vi "(Depricated) EnQ Syringe Pressure State.vi"(6 "Raw Pressure":dbl=nan, 7 "d/dt":dbl, 8 "error in (no error)":errorcluster, 9 "Pressure":dbl=nan, 10 "State":T1, 11 "cRIO Vacuum in":refnum<class "cRIO Vacuum.lvclass">) -> (0 "error out":errorcluster, 1 "overflow?":bool, 2 "Overflow State":T1, 3 "cRIO Vacuum out":refnum<class "cRIO Vacuum.lvclass">, 4 "Overflow Pressure":dbl, 5 "overflow d/dt":dbl)   [LabVIEW 2015]
uses:
  Controls/Vacuum State Enumerator.ctl
  Controls/Vacuum State Cluster.ctl
  cRIO Vacuum.lvclass
panel:
  out "Overflow Raw Pressure":dbl
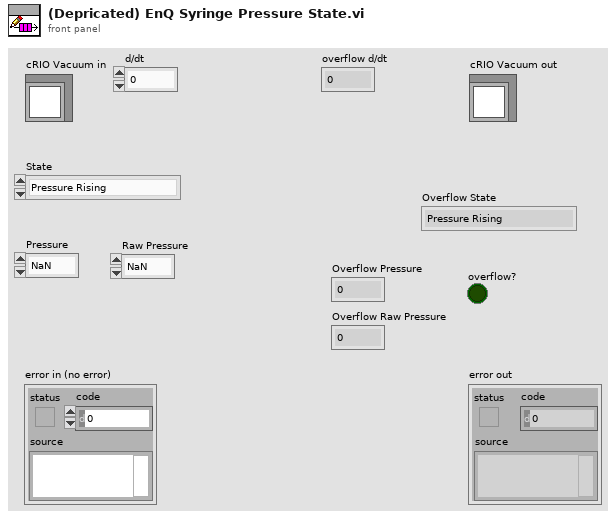
[diagram p1: front panel]
types:
  T1 = typedef "Vacuum State Enumerator.ctl" = enum16{"Pressure Rising", "Plateau", "Pressure Dropping", "Valley", "Low Valley", "Leak", "Unknown"}
  T2 = typedef "Vacuum State Cluster.ctl" = cluster{"Vacuum State":T1, "Pressure":dbl, "Raw Pressure":dbl, "d/dt":dbl}
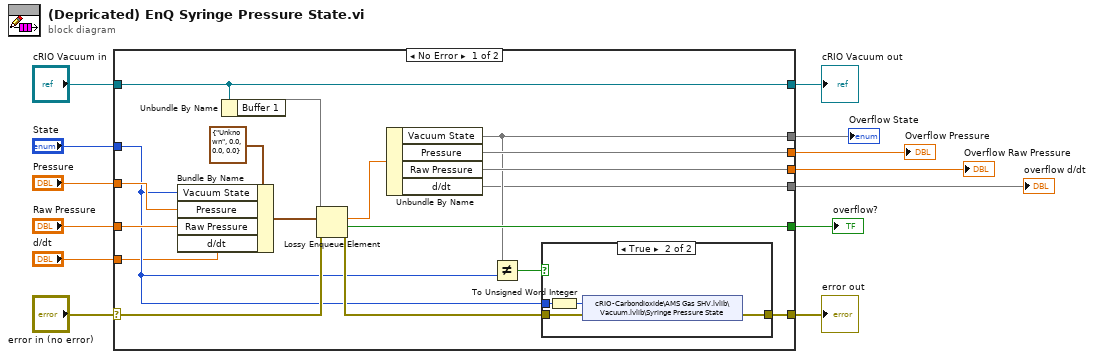
[diagram p0: block diagram]
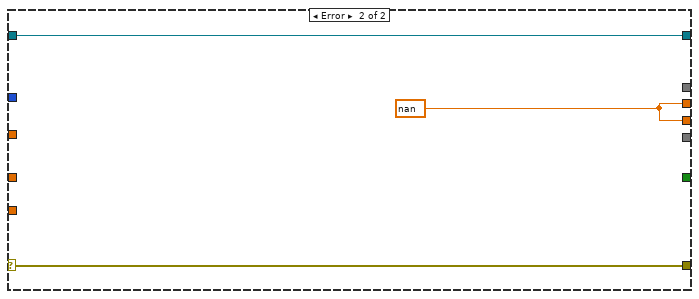
[diagram p3: hidden frame]
diagram:
  n1 = case shown="No Error" "error in (no error)" {
    selector: "error in (no error)" -> [w30 w38]
    tunnel: [w21 w38] -> w12
    tunnel: [w31 w39] -> w10
    tunnel: "cRIO Vacuum in" -> [w31 w39]
    tunnel: "State" -> [w19 _]
    tunnel: [w23 _] -> w8
    tunnel: [w29 _] -> w7
    tunnel: "Pressure" -> [w25 _]
    tunnel: [w27 w37] -> w5
    tunnel: "Raw Pressure" -> [w26 _]
    tunnel: [w24 w37] -> w3
    tunnel: "d/dt" -> [w15 _]
    tunnel: [w14 _] -> w1
    frame No Error {
      n2 = Bundle By Name(cluster=T2 {"Vacuum State"=enum."Unknown", "Pressure"=0.0, "Raw Pressure"=0.0, "d/dt"=0.0} ("element"), "Vacuum State"=w19, "Pressure"=w25, "Raw Pressure"=w26, "d/dt"=w15) -> (w16:T2)
      n3 = Unbundle By Name(w31) -> ("Buffer 1"=w18)
      n4 = Lossy Enqueue Element(queue=w18, element=w16, error in (no error)=w30) -> (overflow element=w28:dbl, overflow?=w29:bool, error out=w22:errorcluster)  [unwired: 1 out]
      n5 = Unbundle By Name(w28) -> ("Vacuum State"=w23, "Pressure"=w27, "Raw Pressure"=w24, "d/dt"=w14)
      n6 = Not Equal?(x=w23, y=w19) -> (x != y?=w20:bool)
      n7 = case shown="True" w20 {
        tunnel: w22 -> [w32 w36]
        tunnel: [w32 w35] -> w21
        tunnel: w19 -> [_ w34]
        frame False {
        }
        frame True {
          n8 = To Unsigned Word Integer(number=w34) -> (unsigned 16bit integer=w33:u16)
          n9 = shared-variable "cRIO-Carbondioxide\\AMS Gas SHV.lvlib\\Vacuum.lvlib\\Syringe Pressure State"(w33, error in=w36) -> (error out=w35:errorcluster)
        }
      }
    }
    frame Error {
      w37 = nan ("Pressure")
    }
  }
  "error out" <- w12
  "cRIO Vacuum out" <- w10
  "Overflow State" <- w8
  "overflow?" <- w7
  "Overflow Pressure" <- w5
  "Overflow Raw Pressure" <- w3
  "overflow d/dt" <- w1
